vi "Set-Jog-Params.vi"(7 "clic IN":dbl min=0.0 max=30.0 step=0.1 format="%.1f") -> (8 "clic OUT":dbl min=0.0 max=30.0 step=0.1 format="%.1f")   [LabVIEW 2011]
panel:
  in  "undo":bool
  in  "accept":bool
  in  "Arcsec/clic":dbl min=0.0 max=30.0 step=0.1 format="%.1f"
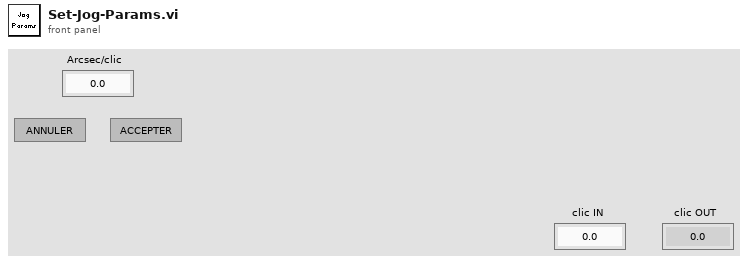
[diagram p1: front panel]
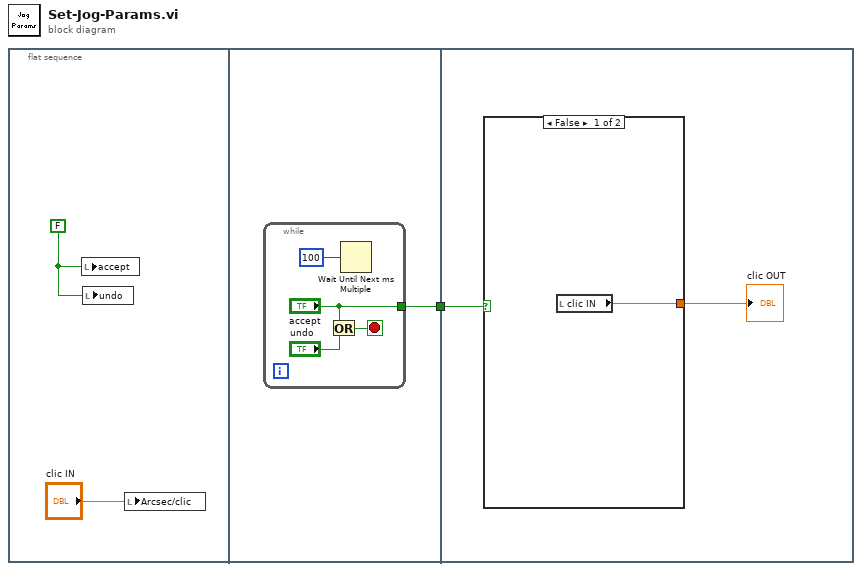
[diagram p0: block diagram]
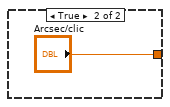
[diagram p2: hidden frame]
diagram:
  n1 = flat-sequence {
    tunnel: [w4] -> w1
    tunnel: w1 -> [w10]
    frame #0 {
      w3 = FALSE
      n2 = local write "accept"(w3) -> ()
      n3 = local write "undo"(w3) -> ()
      n4 = local write "Arcsec/clic"("clic IN") -> ()
    }
    frame #1 {
      n5 = while {
        tunnel: ["accept"] -> w4
        stop <- w6 stop-if-true
        n6 = Or(x="accept", y="undo") -> (x .or. y?=w6:bool)
        n7 = Wait Until Next ms Multiple(millisecond multiple=u32 100 ("milliseconds to wait")) -> ()  [unwired: 1 out]
      }
    }
    frame #2 {
      n8 = case shown="False" w10 {
        tunnel: [w11 "Arcsec/clic"] -> w9
        frame False {
          n9 = local read "clic IN"() -> (w11:dbl)
        }
        frame True {
        }
      }
      "clic OUT" <- w9
    }
  }
